vi "Teardown.vi"(11 "Base Queue jettl in":refnum<class "Base Queue jettl.lvclass">) -> (3 "Base Queue jettl out":refnum<class "Base Queue jettl.lvclass">)   [LabVIEW 2021, in "jettl.lvlib" / "Base Queue jettl.lvlib" / "Base Queue jettl.lvclass"]
uses:
  Base Queue jettl.lvclass
  State/Teardown State/Teardown State.lvclass
  C:/git/jettl/src/jettl/jettl/Base Queue jettl/State/State/State.lvclass
  Base Queue jettl.lvclass/Base Queue jettl.ctl
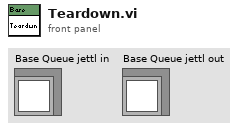
[diagram p1: front panel]
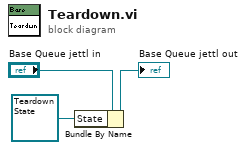
[diagram p0: block diagram]
diagram:
  n1 = Bundle By Name(cluster="Base Queue jettl in", "State"=refnum<class "Teardown State.lvclass"> refnum ("jettl.lvlib:Teardown Queue State.lvclass")) -> (→"Base Queue jettl out":refnum<class "Base Queue jettl.lvclass">)
